vi "PLC-Close.vi"(8 "error in":errorcluster, 11 "Idx":i32) -> (0 "error out":errorcluster)   [LabVIEW 2016]
uses:
  PLC.Action.ctl
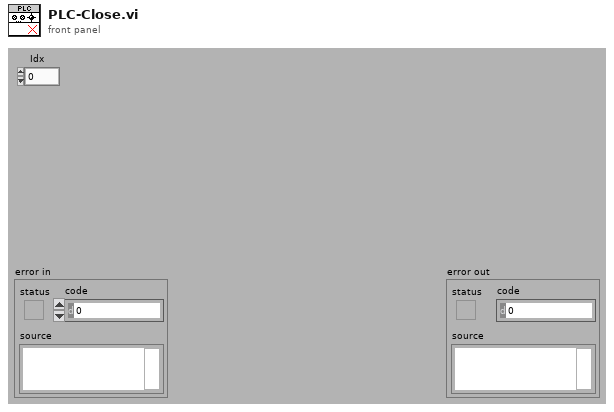
[diagram p1: front panel]
types:
  T1 = typedef "PLC.Action.ctl" = enum32{"idle", "constructor", "destructor", "-- PLC --", "Setup", "NewData", "ChangeOver", "CheckStatus", "Reasembly"}
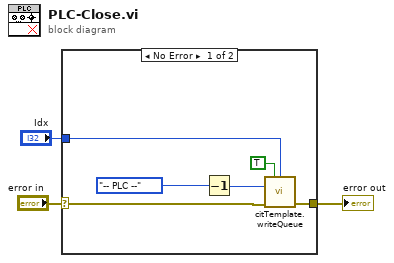
[diagram p0: block diagram]
diagram:
  n1 = case shown="No Error" "error in" {
    selector: "error in" -> [w8 w10]
    tunnel: [w7 w10] -> w2
    tunnel: "Idx" -> [w4 _]
    frame No Error {
      n2 = Decrement(x=PLC.Action."-- PLC --" ("Action")) -> (x-1=w6:T1)
      n3 = call "citTemplate.writeQueue.vi"("High priority (F)"=TRUE, "instance (0)"=w4, "event in (if not connected:all statemachine with data event)"=w6, "error in (no error)"=w8) -> ("error out"=w7:errorcluster)  [unwired: 11 in]
    }
    frame Error {
    }
  }
  "error out" <- w2
